vi "Create.vi"(5 "fifo options":T1, 7 "id (0)":i32, 8 "error in (no error)":errorcluster, 9 "fifo depths (10)":u32=10, 11 "Plugin Interface type":refnum<class "Plugin Interface.lvclass">) -> (0 "error out":errorcluster, 3 "Plugin Interface":refnum<class "Plugin Interface.lvclass">)   [LabVIEW 2021, in "DSF Core.lvlib" / "Plugin Interface.lvclass"]
uses:
  Plugin Interface.lvclass
  C:/dev/git/custom-devices/niveristand-data-sharing-framework-custom-device/Source/Core/Classes/Interface/Interface.lvclass
  Typedefs/DSF FIFO Options.ctl
  Response Data.ctl
  Response.ctl
  Response Parameters.ctl
  Command Data.ctl
  Command.ctl
  Command Parameters.ctl
  FIFO Descriptors.ctl
  FIFO Descriptor.ctl
  Interface.lvclass/Interface.ctl
  Create RT FIFO.vi
  Interface.lvclass
  Framework/Framework.lvclass
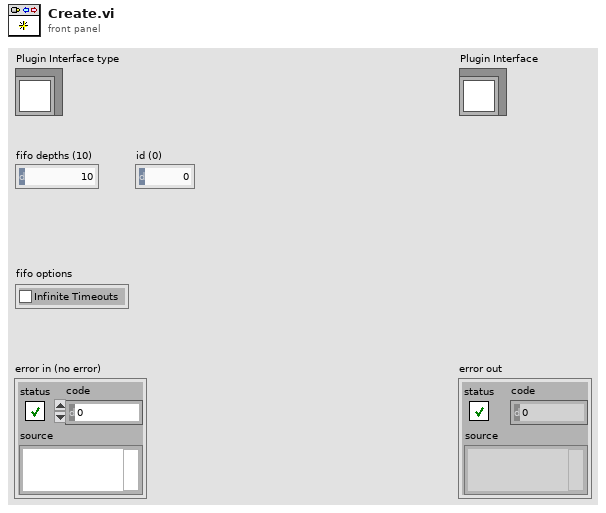
[diagram p1: front panel]
types:
  T1 = typedef "DSF Core.lvlib/Framework.lvclass/DSF FIFO Options.ctl" = cluster{"Infinite Timeouts":bool}
  T2 = typedef "DSF Core.lvlib/Plugin Interface.lvclass/Response Data.ctl" = cluster{"Response":T3, "Parameters":T4}
  T3 = typedef "DSF Core.lvlib/Plugin Interface.lvclass/Response.ctl" = enum8{"General Ack", "Shutting Down"}
  T4 = typedef "DSF Core.lvlib/Plugin Interface.lvclass/Response Parameters.ctl" = cluster{"arg1":u64, "arg2":u64}
  T5 = typedef "DSF Core.lvlib/Plugin Interface.lvclass/Command Data.ctl" = cluster{"Command":T6, "Parameters":T7}
  T6 = typedef "DSF Core.lvlib/Plugin Interface.lvclass/Command.ctl" = enum8{"Idle", "Start", "Set Inline Buffer", "Rx", "Tx", "Shutdown", "Error"}
  T7 = typedef "DSF Core.lvlib/Plugin Interface.lvclass/Command Parameters.ctl" = cluster{"arg1":u64, "arg2":u64}
  T8 = typedef "DSF Core.lvlib/Interface.lvclass/FIFO Descriptors.ctl" = cluster{"command fifo":T9, "response fifo":T9, "error fifo":T9}
  T9 = typedef "DSF Core.lvlib/Interface.lvclass/FIFO Descriptor.ctl" = cluster{"fifo depth":u32, "element size":u32}
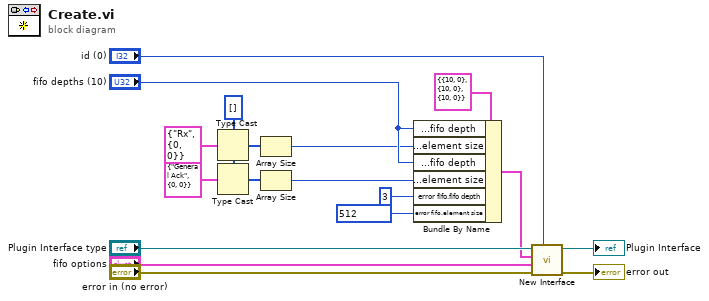
[diagram p0: block diagram]
diagram:
  w2 = u8[] [] ("element")
  n1 = Type Cast(type=w2, x=T5 {"Command"=enum."Rx", "Parameters"={"arg1"=0, "arg2"=0}} ("Plugin Command")) -> (*(type *) &x=w8:u8[])
  n2 = Type Cast(type=w2, x=T2 {"Response"=enum."General Ack", "Parameters"={"arg1"=0, "arg2"=0}} ("Plugin Response")) -> (*(type *) &x=w6:u8[])
  n3 = Array Size(array=w8) -> (size(s)=w7:i32)
  n4 = Array Size(array=w6) -> (size(s)=w4:i32)
  n5 = Bundle By Name(cluster=T8 {"command fifo"={"fifo depth"=10, "element size"=0}, "response fifo"={"fifo depth"=10, "element size"=0}, "error fifo"={"fifo depth"=10, "element size"=0}} ("fifo descriptors"), "command fifo.fifo depth"="fifo depths (10)", "command fifo.element size"=w7, "response fifo.fifo depth"="fifo depths (10)", "response fifo.element size"=w4, "error fifo.fifo depth"=u32 3, "error fifo.element size"=u32 512 ("element size")) -> (w13:T8)
  n6 = call "New Interface.vi"("id (0)"="id (0)", "error in (no error)"="error in (no error)", "fifo options"="fifo options", "fifo descriptors"=w13, "Interface type"="Plugin Interface type") -> ("error out"=→"error out":errorcluster, "Interface"=→"Plugin Interface":refnum<class "Plugin Interface.lvclass">)  [unwired: 5 in]
